vi "Initialize Results.vi"(8 "error in (no error)":errorcluster, 11 "Application in":refnum<class "Application.lvclass">) -> (0 "error out":errorcluster, 3 "Application out":refnum<class "Application.lvclass">)   [LabVIEW 2017, in "Application.lvlib" / "Application.lvclass"]
doc: "Clears out the local data of 'results'. Loads it with an Empty Fail Code, Passing Result, and the correct position. Should only be used prior to the beginning of a test."
uses:
  Application.lvclass
  Application.lvclass/Application.ctl
  Properties/Test Result -- Cluster.ctl
  Properties/App Properties.lvclass
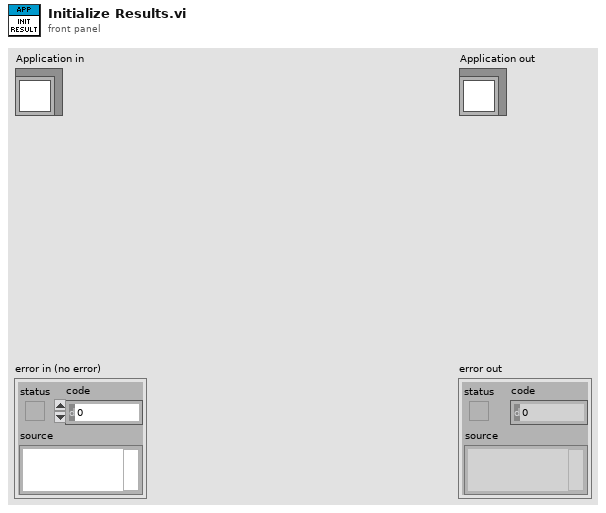
[diagram p1: front panel]
types:
  T1 = cluster{"Serial Number Reference":refnum<vi>, "Status Message Reference":refnum<vi>, "Position":u32}[]
  T2 = typedef "Application.lvlib/App Properties.lvclass/Test Result -- Cluster.ctl" = cluster{"Position":i32, "Pass":bool, "Fail Codes":string}
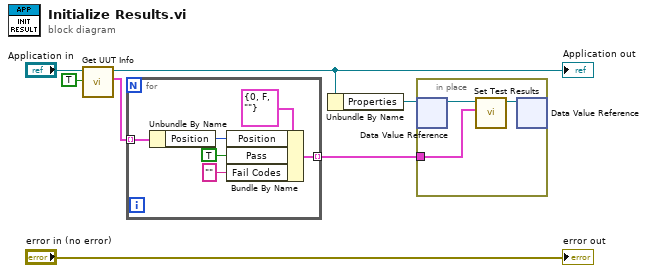
[diagram p0: block diagram]
diagram:
  n1 = call-dynamic "Get UUT Info.vi"("Scanned Only (false)"=TRUE, "Application in"="Application in") -> ("All UUTs"=w2:T1, "Application out"=w3:refnum<class "Application.lvclass">)  [unwired: 7 in, 1 out]
  "Application out" <- w3
  n2 = for {
    tunnel: w2 -> [w13] mode=indexing
    tunnel: [w10] -> w5 mode=indexing
    n3 = Unbundle By Name(w13) -> ("Position"=w11:u32)
    n4 = Bundle By Name(cluster=T2 {"Position"=0, "Pass"=FALSE, "Fail Codes"=""} ("Test Results"), "Position"=w11, "Pass"=TRUE, "Fail Codes"="") -> (w10:T2)
  }
  n5 = Unbundle By Name(w3) -> ("Properties"=w6:refnum<data-value>)
  n6 = in-place {
    in-place-border: w5 -> [w14]
    n7 = in-place-dvr #1(w6) -> (w16:refnum<class "App Properties.lvclass">)  [unwired: 1 out]
    n8 = call-dynamic "Set Test Results.vi"("Test Results"=w14, "App Properties in"=w16) -> ("App Properties out"=w15:refnum<class "App Properties.lvclass">)  [unwired: 8 in, 1 out]
    n9 = in-place-dvr #1(w15) -> ()  [unwired: 2 out]
  }
  "error out" <- "error in (no error)"
